vi "Fix_Buscoords.vi"(8 "error in (no error)":errorcluster, 10 "Avoid screen ratio":bool, 11 "BusCoords Path":path) -> (0 "error out":errorcluster, 2 "New positions":cluster{"X":i32, "Y":i32}[](array[cluster]), 3 "Bus_Name":string[](array[string]), 4 "Max X":i32, 6 "Max Y":i32)   [LabVIEW 2010]
doc: "This Vi fixes the buscoords delivered by the user to be compatible with the DSSim-PC GUI.\n\nCreated by Davis Montenegro\n20-10-2014"
uses:
  Vars/Global_Pictures.vi
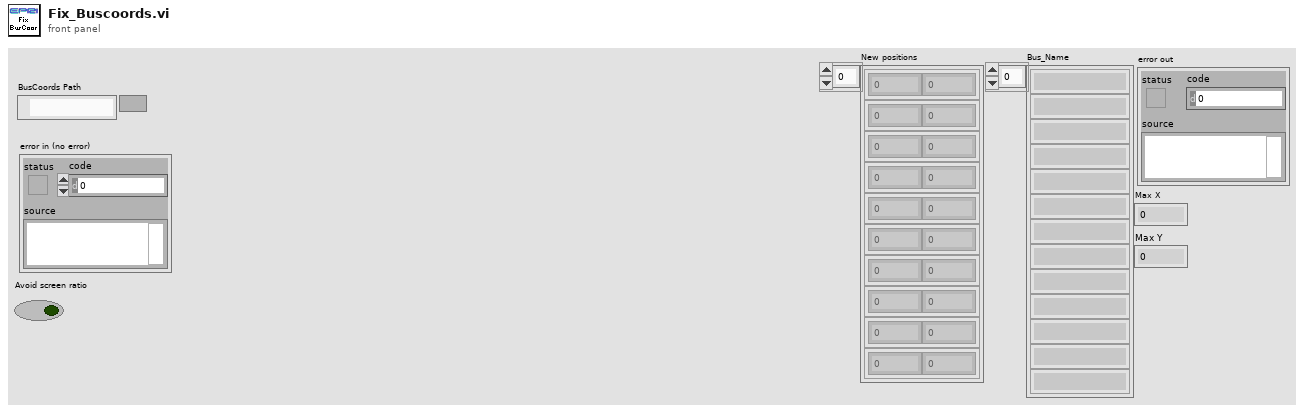
[diagram p1: front panel]
types:
  T1 = typedef "LVBoundsTypeDef.ctl" = cluster{"Width":u32, "Height":u32}
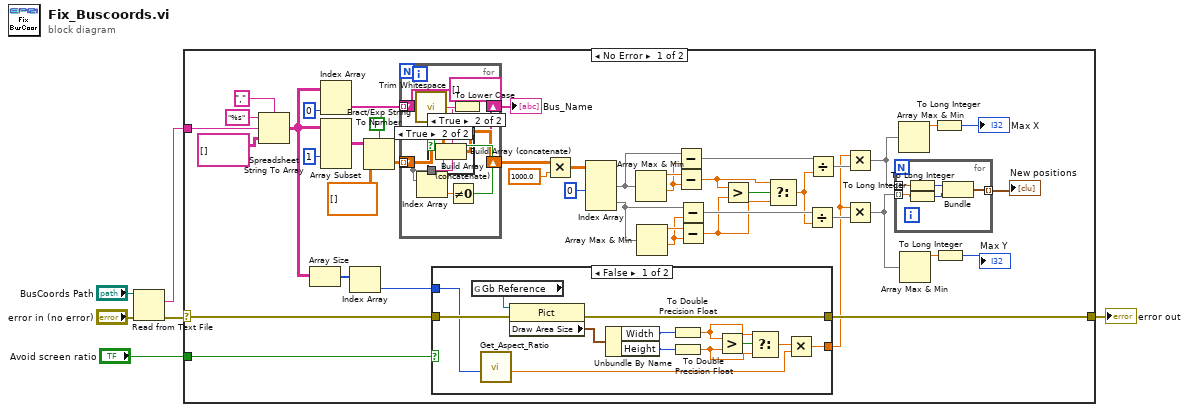
[diagram p0: block diagram]
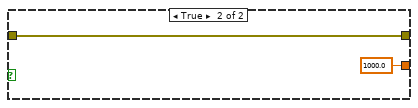
[diagram p2: hidden frame]
diagram:
  n1 = Read from Text File(file (use dialog)="BusCoords Path", error in="error in (no error)") -> (text=w6:string, error out=w3:errorcluster)  [unwired: 2 in, 2 out]
  n2 = case shown="No Error" w3 {
    selector: w3 -> [w24 w90]
    tunnel: w6 -> [w49 _]
    tunnel: [w23 w90] -> w2
    tunnel: "Avoid screen ratio" -> [w15 _]
    frame No Error {
      n3 = Spreadsheet String To Array(delimiter (Tab)=",", format string="%s", spreadsheet string=w49, array type (2D Dbl)=string[][] []) -> (array=w11:string[][])
      n4 = Array Size(array=w11) -> (size(s)=w10:i32[])
      n5 = Index Array(array=w11, index (col)=0 ("disabled index (col)")) -> (element=w41:string[])  [unwired: 1 in]
      n6 = Array Subset(array=w11, index (col)=1 ("index")) -> (w46:string[][])  [unwired: 3 in]
      n7 = Index Array(array=w10) -> (element=w9:i32)  [unwired: 1 in]
      n8 = Fract/Exp String To Number(use system decimal point (T)=FALSE, string=w46) -> (number=w44:dbl[][])  [unwired: 2 in, 1 out]
      n9 = for {
        tunnel: w44 -> [w80] mode=indexing
        tunnel: w41 -> [w78] mode=indexing
        shift-right: [w74] -> w27
        shift-left: dbl[][] [] ("Array") -> [w75]
        shift-right: [w72] -> w40
        shift-left: string[] [] ("Array") -> [w73]
        n10 = call <vilib>:"Trim Whitespace.vi"("string"=w78) -> ("trimmed string"=w77:string)  [unwired: 1 in]
        n11 = Index Array(array=w80) -> (element=w81:dbl)  [unwired: 1 in]
        n12 = Not Equal To 0?(x=w81) -> (x != 0?=w79:bool)
        n13 = case shown="True" w79 {
          tunnel: w75 -> [w86 w88]
          tunnel: w80 -> [_ w87]
          tunnel: [w86 w89] -> w74
          frame False {
          }
          frame True {
            n14 = Build Array (concatenate)(w88, w87) -> (w89:dbl[][])
          }
        }
        n15 = To Lower Case(string=w77) -> (all lower case string=w76:string)
        n16 = case shown="True" w79 {
          tunnel: w73 -> [w82 w84]
          tunnel: w76 -> [_ w83]
          tunnel: [w82 w85] -> w72
          frame False {
          }
          frame True {
            n17 = Build Array (concatenate)(w84, w83) -> (w85:string[])
          }
        }
      }
      "Bus_Name" <- w40
      n18 = case shown="False" w15 {
        tunnel: w24 -> [w64 w65]
        tunnel: [w61 w65] -> w23
        tunnel: [w54 1000.0] -> w16
        tunnel: w9 -> [w53 _]
        frame False {
          n19 = global read "Global_Pictures.vi" "Gb Reference"() -> (w63:refnum<vi>)
          n20 = call "Get_Aspect_Ratio.vi"("# Buses"=w53) -> ("Aspect ratio"=w52:dbl)  [unwired: 10 in]
          n21 = property class="Pict"(reference=w63, error in=w64) -> (error out=w61:errorcluster, "Draw Area Size"=w62:T1)  [unwired: 1 out]
          n22 = Unbundle By Name(w62) -> ("Width"=w60:u32, "Height"=w59:u32)
          n23 = To Double Precision Float(number=w60) -> (double precision float=w56:dbl)
          n24 = To Double Precision Float(number=w59) -> (double precision float=w57:dbl)
          n25 = Greater?(x=w56, y=w57) -> (0:w58:bool)
          n26 = Select(t=w56, s=w58, f=w57) -> (s? t:f=w55:dbl)
          n27 = Multiply(x=w55, y=w52) -> (x*y=w54:dbl)
        }
        frame True {
        }
      }
      n28 = Multiply(x=w27, y=1000.0) -> (x*y=w26:dbl[][])
      n29 = Index Array(array=w26, index (col) #1=0 ("disabled index (col)")) -> (element #1=w35:dbl[], element #2=w30:dbl[])  [unwired: 3 in]
      n30 = Array Max & Min(array=w35) -> (max value=w34:dbl, min value=w33:dbl)  [unwired: 2 out]
      n31 = Array Max & Min(array=w30) -> (max value=w31:dbl, min value=w29:dbl)  [unwired: 2 out]
      n32 = Subtract(x=w35, y=w33) -> (x-y=w32:dbl[])
      n33 = Subtract(x=w34, y=w33) -> (x-y=w20:dbl)
      n34 = Subtract(x=w30, y=w29) -> (x-y=w28:dbl[])
      n35 = Subtract(x=w31, y=w29) -> (x-y=w19:dbl)
      n36 = Greater?(x=w20, y=w19) -> (0:w17:bool)
      n37 = Select(t=w20, s=w17, f=w19) -> (s? t:f=w18:dbl)
      n38 = Divide(x=w28, y=w18) -> (x/y=w21:dbl[])
      n39 = Divide(x=w32, y=w18) -> (x/y=w22:dbl[])
      n40 = Multiply(x=w16, y=w22) -> (x*y=w39:dbl[])
      n41 = Multiply(x=w16, y=w21) -> (x*y=w13:dbl[])
      n42 = for {
        tunnel: w39 -> [w71] mode=indexing
        tunnel: w13 -> [w69] mode=indexing
        tunnel: [w67] -> w43 mode=indexing
        n43 = To Long Integer(number=w71) -> (32bit integer=w70:i32)
        n44 = To Long Integer(number=w69) -> (32bit integer=w68:i32)
        n45 = Bundle(w70, w68) -> (w67:cluster{i32, i32})  [unwired: 1 in]
      }
      "New positions" <- w43
      n46 = Array Max & Min(array=w39) -> (max value=w38:dbl)  [unwired: 3 out]
      n47 = Array Max & Min(array=w13) -> (max value=w14:dbl)  [unwired: 3 out]
      n48 = To Long Integer(number=w38) -> (32bit integer=→"Max X":i32)
      n49 = To Long Integer(number=w14) -> (32bit integer=→"Max Y":i32)
    }
    frame Error {
    }
  }
  "error out" <- w2
